vi "readTelemetryAirData.vi"(8 "error in (no error)":errorcluster, 10 "Parser":refnum<class "U8ArrayParserAutoIndexing.lvclass">, 11 "M1M3SAL in":refnum<class "M1M3SAL.lvclass">) -> (0 "error out":errorcluster, 2 "EventSummaryState":variant, 3 "M1M3SAL out":refnum<class "M1M3SAL.lvclass">)   [LabVIEW 2016, in "M1M3SupportCommunicator.lvlib" / "M1M3SAL.lvclass"]
uses:
  M1M3SAL.lvclass
  Common_RT_Utilities/U8ArrayParserAutoIndexing/U8ArrayParserAutoIndexing.lvclass
  DataTypes/Topics/TelemetryAirData.ctl
  DataTypes/Topics/Parts/Timestamp.ctl
  DataTypes/Topics/M1M3SupportTopics.lvlib
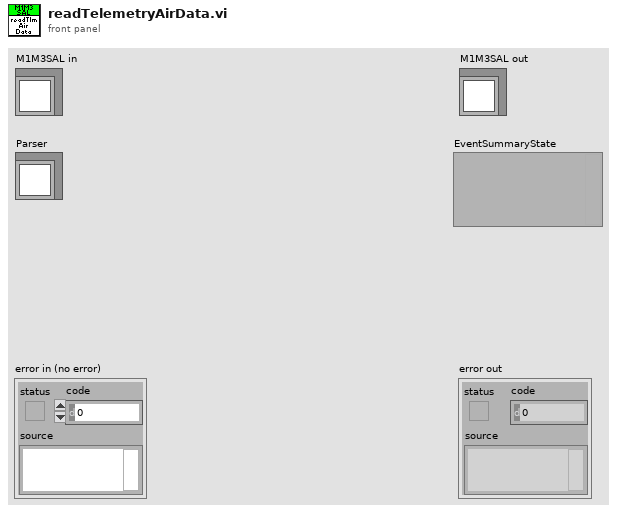
[diagram p1: front panel]
types:
  T1 = typedef "M1M3SupportTopics.lvlib/TelemetryAirData.ctl" = cluster{"Timestamp":T2, "CellAirPressure":sgl, "HardpointAirPressure":sgl}
  T2 = typedef "M1M3SupportTopics.lvlib/Timestamp.ctl" = dbl
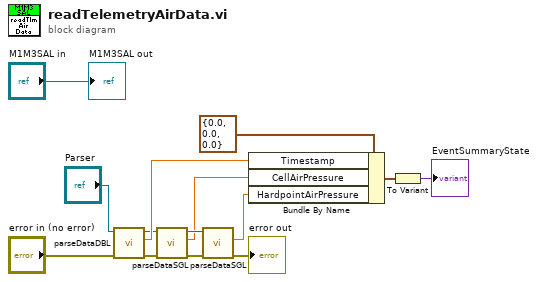
[diagram p0: block diagram]
diagram:
  n1 = call "parseDataDBL.vi"("error in (no error)"="error in (no error)", "U8ArrayParserAutoIndexing in"="Parser") -> ("error out"=w5:errorcluster, "Data"=w9:dbl, "U8ArrayParserAutoIndexing out"=w7:refnum<class "U8ArrayParserAutoIndexing.lvclass">)  [unwired: 7 in]
  n2 = call "parseDataSGL.vi"("error in (no error)"=w5, "U8ArrayParserAutoIndexing in"=w7) -> ("error out"=w4:errorcluster, "Data"=w2:sgl, "U8ArrayParserAutoIndexing out"=w6:refnum<class "U8ArrayParserAutoIndexing.lvclass">)  [unwired: 7 in]
  n3 = call "parseDataSGL.vi"("error in (no error)"=w4, "U8ArrayParserAutoIndexing in"=w6) -> ("error out"=→"error out":errorcluster, "Data"=w1:sgl)  [unwired: 7 in, 1 out]
  n4 = Bundle By Name(cluster=T1 {"Timestamp"=0.0, "CellAirPressure"=0.0, "HardpointAirPressure"=0.0} ("TelemetryAirData"), "Timestamp"=w9, "CellAirPressure"=w2, "HardpointAirPressure"=w1) -> (w13:T1)
  n5 = To Variant(anything=w13) -> (Variant=→"EventSummaryState":variant)
  "M1M3SAL out" <- "M1M3SAL in"
